vi "飞轮控制命令（29）2.vi"(0 "最高转速":dbl, 1 "电机启动控制指令":bool, 5 "力矩最大值(uNm)":dbl, 7 "pwmperiod":dbl, 9 "模式选择":u16(ring) items=["电流校正模式", "转矩模式", "转速模式", "开环测试模式"], 11 "模式确定":bool, 12 "写指令字":dbl) -> (4 "字符串":string)   [LabVIEW 2012]
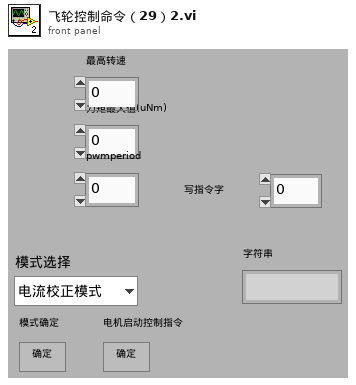
[diagram p1: front panel]
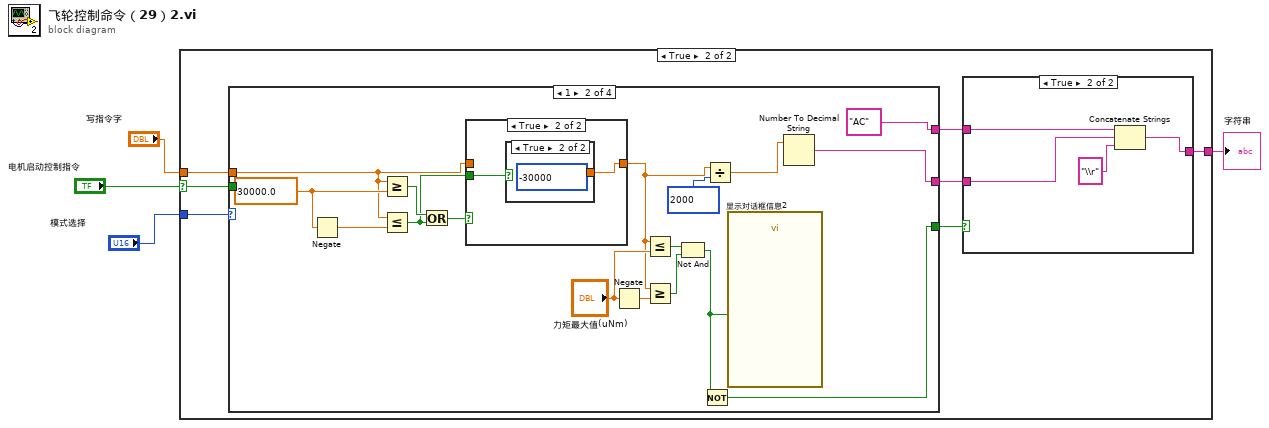
[diagram p0: block diagram]
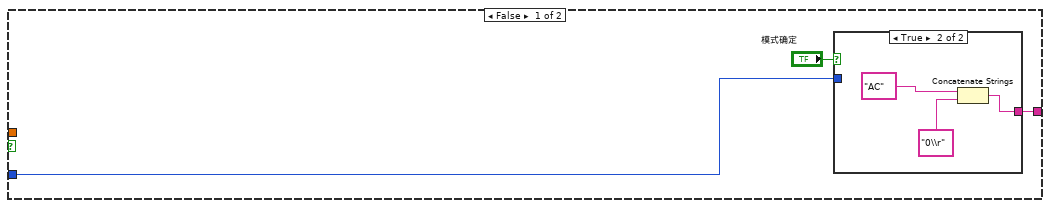
[diagram p2: hidden frame]
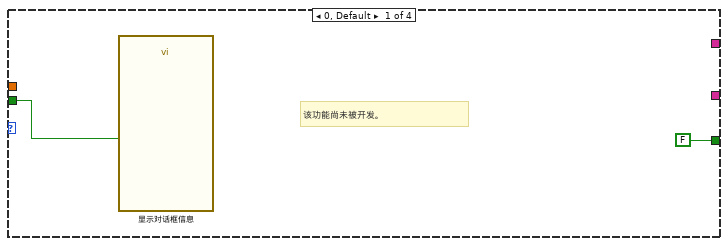
[diagram p5: hidden frame]
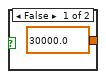
[diagram p7: hidden frame]
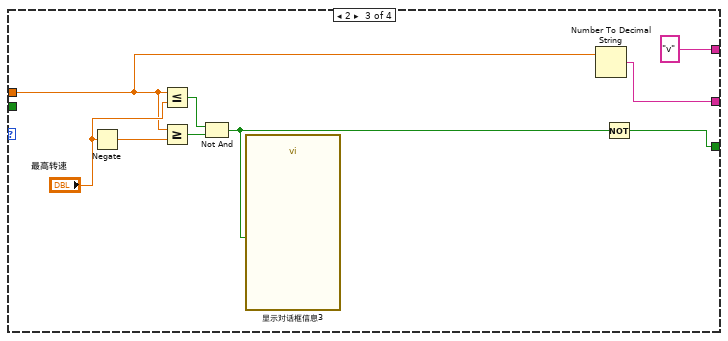
[diagram p8: hidden frame]
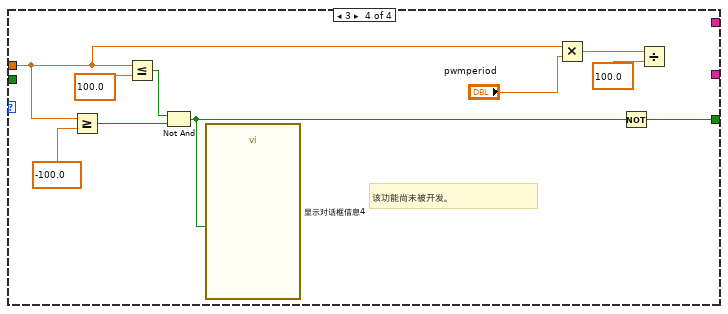
[diagram p9: hidden frame]
diagram:
  n1 = case shown="True" "电机启动控制指令" {
    selector: "电机启动控制指令" -> [_ w16]
    tunnel: "模式选择" -> [w6 w15]
    tunnel: "写指令字" -> [_ w14]
    tunnel: [w5 w13] -> w1
    frame False {
      n2 = case shown="True" "模式确定" {
        tunnel: [_ w9] -> w5
        tunnel: w6 -> [_ _]
        frame False {
        }
        frame True {
          n3 = Concatenate Strings("AC", "0\\r") -> (w9:string)
        }
      }
    }
    frame True {
      n4 = case shown="1" w15 {
        tunnel: [FALSE w37 w51 w56] -> w17
        tunnel: w14 -> [_ w32 w48 w55]
        tunnel: w16 -> [w22 _ _ _]
        tunnel: [_ w24 w47 _] -> w12
        tunnel: [_ "AC" "v" _] -> w11
        frame 0, Default {
          # "该功能尚未被开发。"
          n5 = call "显示对话框信息"("Enable"=w22) -> ()  [unwired: 2 in, 9 out]
        }
        frame 1 {
          w34 = 30000.0 ("x")
          n6 = Negate(x=w34) -> (-x=w33:dbl)
          n7 = Greater Or Equal?(x=w32, y=w34) -> (x >= y?=w31:bool)
          n8 = Less Or Equal?(x=w32, y=w33) -> (x <= y?=w30:bool)
          n9 = Or(x=w31, y=w30) -> (x .or. y?=w29:bool)
          n10 = case shown="True" w29 {
            tunnel: [w41 w42] -> w27
            tunnel: w32 -> [w41 _]
            tunnel: w30 -> [_ w43]
            frame False {
            }
            frame True {
              n11 = case shown="True" w43 {
                tunnel: [30000.0 ("x") -30000] -> w42
                frame False {
                }
                frame True {
                }
              }
            }
          }
          n12 = Negate(x="力矩最大值(uNm)") -> (-x=w36:dbl)
          n13 = Less Or Equal?(x=w27, y="力矩最大值(uNm)") -> (x <= y?=w39:bool)
          n14 = Greater Or Equal?(x=w27, y=w36) -> (x >= y?=w40:bool)
          n15 = Not And(1:w40, 2:w39) -> (0:w38:bool)
          n16 = Not(x=w38) -> (.not. x?=w37:bool)
          n17 = Divide(x=w27, y=2000) -> (x/y=w25:dbl)
          n18 = call "显示对话框信息2"("Enable"=w38) -> ()  [unwired: 2 in, 9 out]
          n19 = Number To Decimal String(number=w25) -> (decimal integer string=w24:string)  [unwired: 1 in]
        }
        frame 2 {
          n20 = Negate(x="最高转速") -> (-x=w49:dbl)
          n21 = Less Or Equal?(x=w48, y="最高转速") -> (x <= y?=w53:bool)
          n22 = Greater Or Equal?(x=w48, y=w49) -> (x >= y?=w54:bool)
          n23 = Not And(1:w54, 2:w53) -> (0:w52:bool)
          n24 = call "显示对话框信息3"("Enable"=w52) -> ()  [unwired: 2 in, 9 out]
          n25 = Number To Decimal String(number=w48) -> (decimal integer string=w47:string)  [unwired: 1 in]
          n26 = Not(x=w52) -> (.not. x?=w51:bool)
        }
        frame 3 {
          # "该功能尚未被开发。"
          n27 = Greater Or Equal?(x=w55, y=-100.0) -> (x >= y?=w64:bool)
          n28 = Less Or Equal?(x=w55, y=100.0) -> (x <= y?=w63:bool)
          n29 = Not And(1:w64, 2:w63) -> (0:w57:bool)
          n30 = call "显示对话框信息4"("Enable"=w57) -> ()  [unwired: 2 in, 9 out]
          n31 = Multiply(x=w55, y="pwmperiod") -> (x*y=w59:dbl)
          n32 = Not(x=w57) -> (.not. x?=w56:bool)
          n33 = Divide(x=w59, y=100.0) -> ()  [unwired: 1 out]
        }
      }
      n34 = case shown="True" w17 {
        tunnel: [_ w19] -> w13
        tunnel: w12 -> [_ w20]
        tunnel: w11 -> [_ w21]
        frame False {
        }
        frame True {
          n35 = Concatenate Strings(w21, w20, "\\r" ("string")) -> (w19:string)
        }
      }
    }
  }
  "字符串" <- w1
